vi "Read Settings.vi"(8 "error in (no error)":errorcluster, 11 "PowerSupply in":refnum<class "PowerSupply.lvclass">) -> (0 "error out":errorcluster, 2 "Settings":T1, 3 "PowerSupply out":refnum<class "PowerSupply.lvclass">)   [LabVIEW 2019, in "PowerSupply.lvlib" / "PowerSupply.lvclass"]
uses:
  Library/PowerSupply.lvclass
  Custom Controls/Settings.ctl
  Custom Controls/OCP Mode.ctl
  Custom Controls/Sense Point.ctl
  Library/PowerSupply.lvclass/PowerSupply.ctl
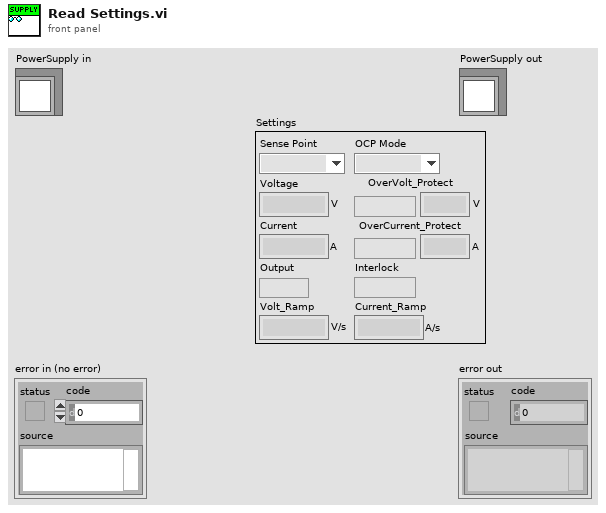
[diagram p1: front panel]
types:
  T1 = typedef "PowerSupply.lvlib/PowerSupply.lvclass/Settings.ctl" = cluster{"Volt_Ramp":dbl, "Output":bool, "Current":dbl, "Voltage":dbl, "Current_Ramp":dbl, "Interlock":bool, "OCP":bool, "OverCurrent_Protect":dbl, "OVP":bool, "OverVolt_Protect":dbl, "OCP Mode":T2, "Sense Point":T3}
  T2 = typedef "PowerSupply.lvlib/PowerSupply.lvclass/OCP Mode.ctl" = enum16{"Shutdown", "Foldback"}
  T3 = typedef "PowerSupply.lvlib/PowerSupply.lvclass/Sense Point.ctl" = enum16{"Local", "Remote"}
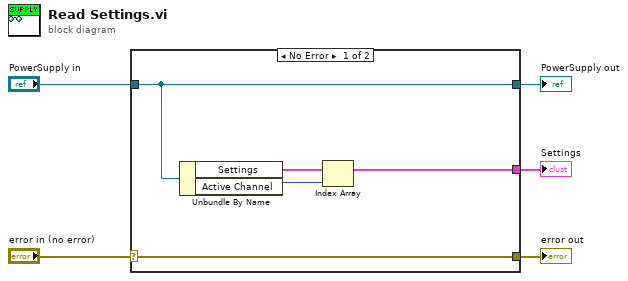
[diagram p0: block diagram]
diagram:
  n1 = case shown="No Error" "error in (no error)" {
    selector: "error in (no error)" -> [w10 w11]
    tunnel: [w10 w11] -> w4
    tunnel: [w9 w12] -> w2
    tunnel: "PowerSupply in" -> [w9 w12]
    tunnel: [w7 _] -> w1
    frame No Error {
      n2 = Unbundle By Name(w9) -> ("Settings"=w8:T1[], "Active Channel"=w6:u32)
      n3 = Index Array(array=w8, index=w6) -> (element=w7:T1)
    }
    frame Error {
    }
  }
  "error out" <- w4
  "PowerSupply out" <- w2
  "Settings" <- w1
